vi "BL132 CAM7 manu.vi"() -> ()   [LabVIEW 2015]
panel:
  out "BL132 MAN":T1(plugin-control)
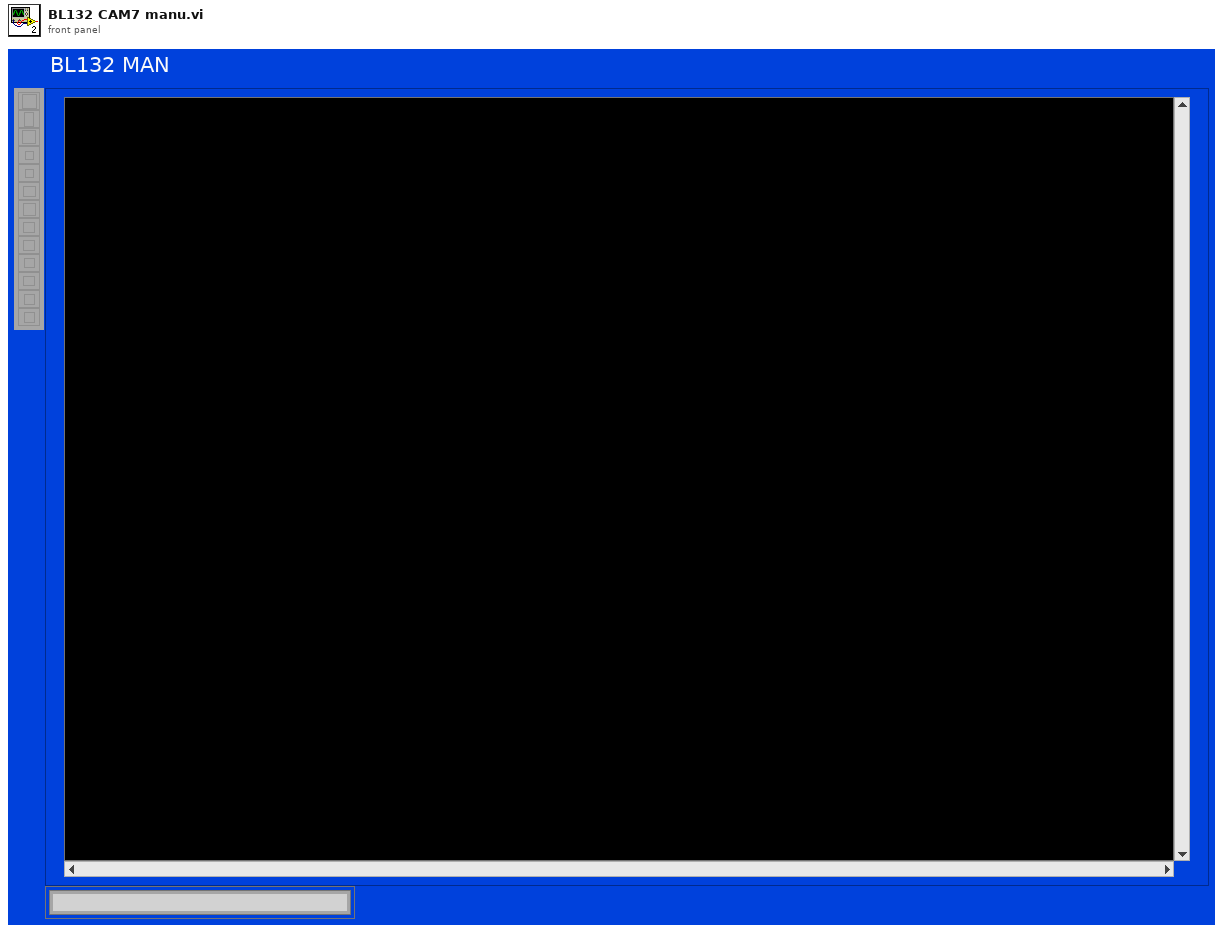
[diagram p1: front panel]
types:
  T1 = typedef "IMAQ Image.ctl" = refnum<image>
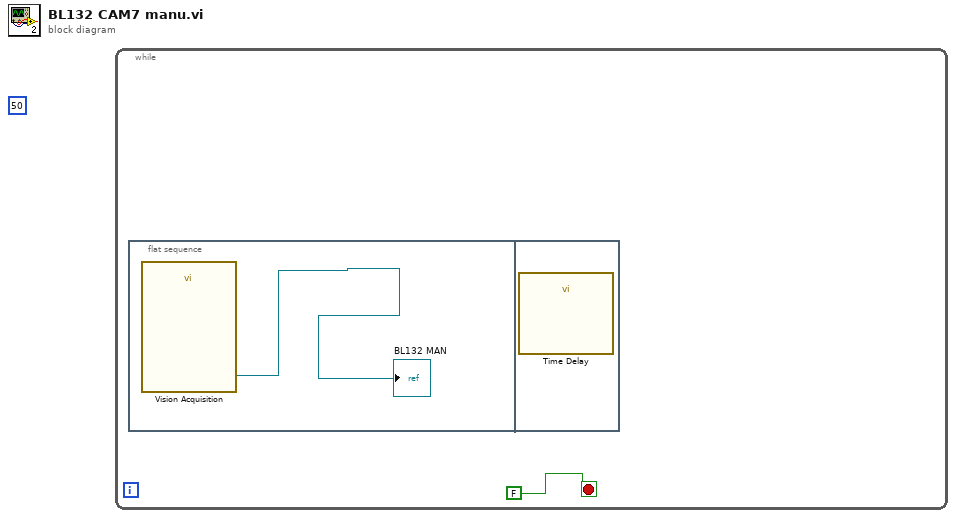
[diagram p0: block diagram]
diagram:
  (unwired) 50 ("Priority")
  n1 = while {
    stop <- FALSE stop-if-true
    n2 = flat-sequence {
      frame #0 {
        n3 = call "Vision Acquisition"() -> ("Image Out"=→"BL132 MAN":T1)  [unwired: 26 in, 1 out]
      }
      frame #1 {
        n4 = call "Time Delay"() -> ()  [unwired: 11 in, 1 out]
      }
    }
  }
